vi "J1939 Address Claim Address.vi"(8 "error in":errorcluster, 9 "Byte Cluster":u8[](array[numeric]), 10 "Requested Address":u8, 11 "Write Session":refnum<k21>) -> (0 "error out":errorcluster, 3 "Write Session out":refnum<k21>)   [LabVIEW 2013, in "J1939.lvlib"]
uses:
  J1939.lvlib
  API Types/CAN Outgoing Message Cluster.ctl
  API Types/PGN Fields Cluster.ctl
  Frame Conversion/Convert J1939 ID to CAN Arb ID.vi
  <vilib>/xnet/xnet.llb/XNET Write (Frame CAN).vi
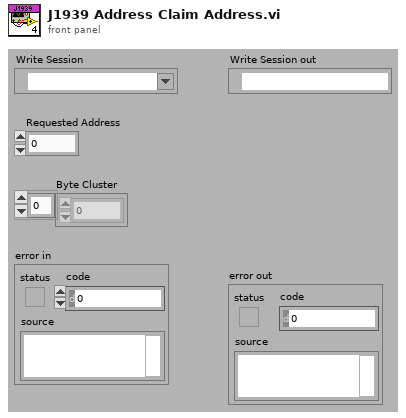
[diagram p1: front panel]
types:
  T1 = typedef "J1939.lvlib/PGN Fields Cluster.ctl" = cluster{"Reserved Bit":u8, "Data page":u8, "PDU Format":u8, "PDU Specific":u8}
  T2 = typedef "J1939.lvlib/CAN Outgoing Message Cluster.ctl" = cluster{"Identifier":u32, "Data":u8[]}
  T3 = typedef "XNET Frame CAN.ctl" = cluster{"timestamp":timestamp, "payload":u8[], "identifier":u32, "type":T4, "extended?":bool, "echo?":bool}
  T4 = typedef "XNET Frame Type CAN.ctl" = u8
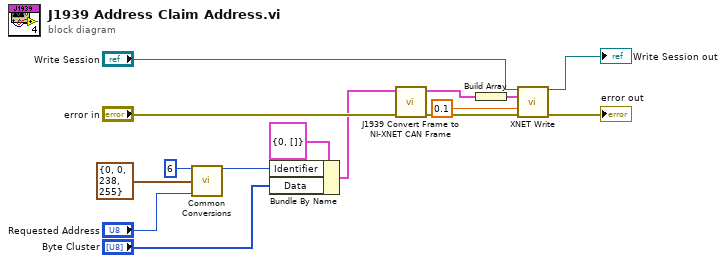
[diagram p0: block diagram]
diagram:
  n1 = call-poly "Common Conversions.vi"("Priority"=u8 6, "PGN Fields"=T1 {"Reserved Bit"=0, "Data page"=0, "PDU Format"=238, "PDU Specific"=255}, "Source Address"="Requested Address") -> ("ID"=w14:u32)  [unwired: 2 in, 10 out]
  n2 = Bundle By Name(cluster=T2 {"Identifier"=0, "Data"=[]} ("Data to Send"), "Identifier"=w14, "Data"="Byte Cluster") -> (w4:T2)
  n3 = call "J1939 Convert Frame to NI-XNET CAN Frame.vi"("error in"="error in", "Data to Send"=w4) -> ("error out"=w5:errorcluster, "CAN frame"=w10:T3)  [unwired: 8 in]
  n4 = Build Array(w10) -> (w1:T3[])
  n5 = call-poly <vilib>:"XNET Write.vi"("session in"="Write Session", "data"=w1, "timeout (10)"=0.1, "error in (no error)"=w5) -> ("session out"=→"Write Session out":refnum<k21>, "error out"=→"error out":errorcluster)  [unwired: 10 out]
